vi "INI Read write String storage.vi"(4 "read/write raw string? (F)":bool, 6 "Values to write":string[](array[string]), 7 "Read/Write mode":T1, 8 "error in":errorcluster, 9 "Defaults":string[](array[string]), 10 "keys":string[](array[string]), 11 "section":string) -> (0 "error out":errorcluster, 2 "Values":string[](array[string]))   [LabVIEW 2013]
doc: "This .vi stores and returns information in the .ini file. It then keeps the latest information in memory. This is an easy way to add .ini functionality to a functional global."
uses:
  Read write mode.ctl
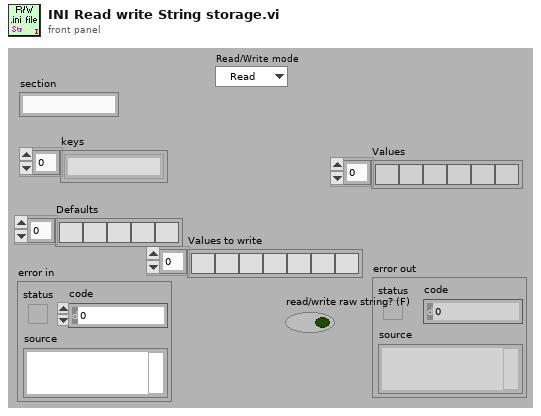
[diagram p1: front panel]
types:
  T1 = typedef "Read write mode.ctl" = enum16{"Read", "Write"}
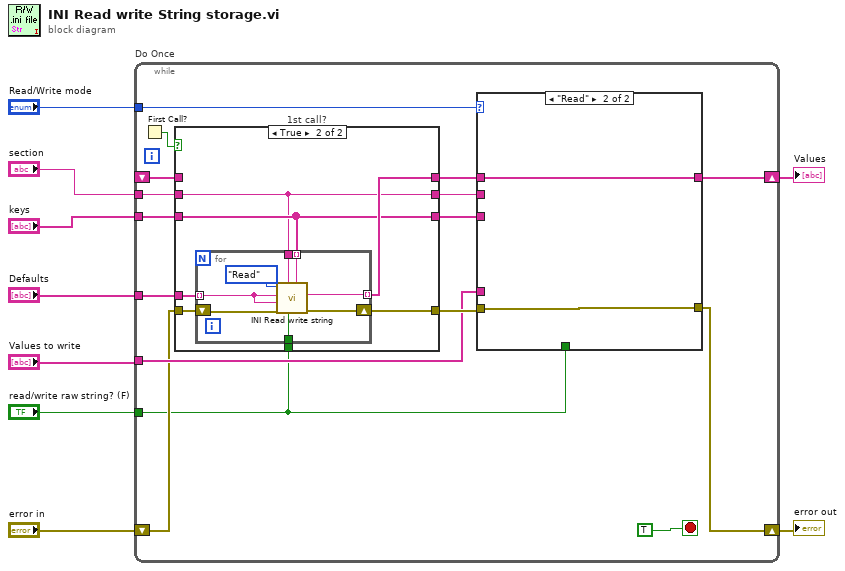
[diagram p0: block diagram]
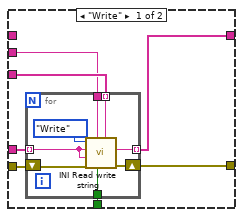
[diagram p2: hidden frame]
diagram:
  n1 = while "Do Once" {
    tunnel: "section" -> [w23]
    tunnel: "Read/Write mode" -> [w22]
    tunnel: "Values to write" -> [w15]
    tunnel: "keys" -> [w17]
    shift-right: [w14] -> w8
    shift-left: _ -> [w16]
    tunnel: "Defaults" -> [w11]
    shift-right: [w12] -> w3
    shift-left: "error in" -> [w13]
    tunnel: "read/write raw string? (F)" -> [w10]
    stop <- TRUE stop-if-true
    n2 = First Call?() -> (First Call?: T/F=w24:bool)
    n3 = case "1st call?" shown="True" w24 {
      tunnel: w23 -> [w46 w49]
      tunnel: w17 -> [w45 w52]
      tunnel: [w44 w53] -> w18
      tunnel: [w43 w48] -> w21
      tunnel: [w46 w49] -> w20
      tunnel: [w45 w52] -> w19
      tunnel: w16 -> [w44 _]
      tunnel: w13 -> [w43 w51]
      tunnel: w11 -> [_ w50]
      tunnel: w10 -> [_ w47]
      frame False {
      }
      frame True {
        n4 = for {
          tunnel: [w60] -> w53 mode=indexing
          shift-right: [w59] -> w48
          shift-left: w51 -> [w61]
          tunnel: w49 -> [w57]
          tunnel: w52 -> [w56] mode=indexing
          tunnel: w50 -> [w55] mode=indexing
          tunnel: w47 -> [w54]
          n5 = call "INI Read write string.vi"("key"=w56, "read/write raw string? (F)"=w54, "section"=w57, "error in"=w61, "Default"=w55, "string in"=w55, "Read|Write"=Read_write_mode."Read") -> ("error out"=w59:errorcluster, "string out"=w60:string)  [unwired: 3 in]
        }
      }
    }
    n6 = case "1st call?" shown="\"Read\"" w22 {
      tunnel: w21 -> [w32 w41]
      tunnel: w20 -> [w28 _]
      tunnel: w19 -> [w31 _]
      tunnel: [w30 w42] -> w14
      tunnel: [w27 w41] -> w12
      tunnel: w18 -> [_ w42]
      tunnel: w15 -> [w29 _]
      tunnel: w10 -> [w26 _]
      frame "Write" {
        n7 = for {
          shift-right: [w39] -> w27
          shift-left: w32 -> [w40]
          tunnel: w31 -> [w37] mode=indexing
          tunnel: w28 -> [w36]
          tunnel: w29 -> [w34] mode=indexing
          tunnel: [w35] -> w30 mode=indexing
          tunnel: w26 -> [w33]
          n8 = call "INI Read write string.vi"("key"=w37, "read/write raw string? (F)"=w33, "section"=w36, "error in"=w40, "Default"=w34, "string in"=w34, "Read|Write"=Read_write_mode."Write") -> ("error out"=w39:errorcluster, "string out"=w35:string)  [unwired: 3 in]
        }
      }
      frame "Read" {
      }
    }
  }
  "Values" <- w8
  "error out" <- w3
